vi "Wait for sync.vi"(8 "error in (no error)":errorcluster, 11 "SyncClient in":refnum<class "SyncClient.lvclass">) -> (0 "error out":errorcluster, 3 "SyncClient out":refnum<class "SyncClient.lvclass">)   [LabVIEW 2020, in "Instrument.lvlib" / "SyncClient.lvclass"]
uses:
  SyncClient.lvclass
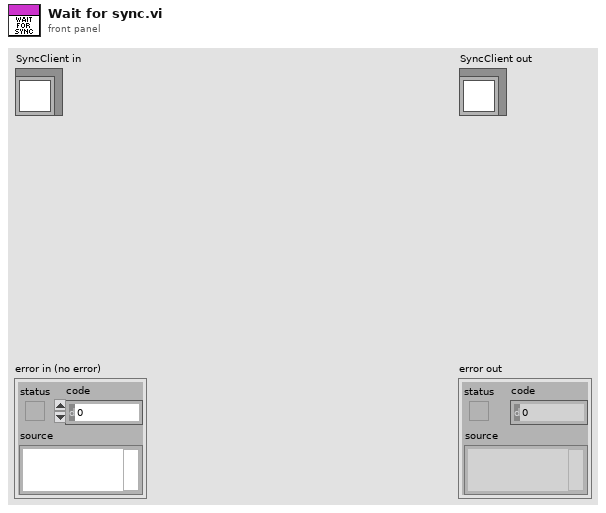
[diagram p1: front panel]
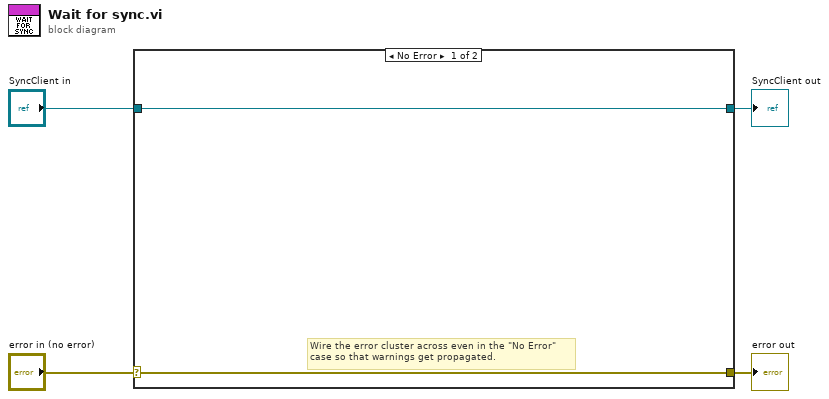
[diagram p0: block diagram]
diagram:
  n1 = case shown="No Error" "error in (no error)" {
    selector: "error in (no error)" -> [w5 w8]
    tunnel: [w5 w8] -> w3
    tunnel: [w6 w7] -> w1
    tunnel: "SyncClient in" -> [w6 w7]
    frame No Error {
      # "Wire the error cluster across even in the \"No Error\"\ncase so that warnings get propagated."
    }
    frame Error {
    }
  }
  "error out" <- w3
  "SyncClient out" <- w1
